vi "filter.post.state.vi"(11 "filter.data in":T1 {"memory.command"."order.slot.value"."Quantity" format="%016x"; "memory.command"."order.slot.value"."OrderId" format="%016x"; "memory.command"."ticker.slot.value"."Symbol" format="%016x"; "Scratch"."OrderId" format="%016x"}) -> (3 "filter.data out 2":T1 {"memory.command"."order.slot.value"."Quantity" format="%016x"; "memory.command"."order.slot.value"."OrderId" format="%016x"; "memory.command"."ticker.slot.value"."Symbol" format="%016x"; "Scratch"."OrderId" format="%016x"})   [LabVIEW 2022 SP3]
uses:
  filter.data.ctl
  filter.states.ctl
  filter.debug.ctl
  filter.debug.slot.ctl
  filter.data.scratch.ctl
  arty/orderbook/orderbook.command.ctl
  arty/orderbook/orderbook.command.type.ctl
  filter.memory.command.ctl
  ticker.slot.ctl
  order.slot.ctl
  <vilib>/rvi/DataTransferAndStorage/Container/Common/niFpgaContainerGetUniqueNameForEmu.vi
  <vilib>/rvi/DataTransferAndStorage/Container/Common/niFpgaContainerSetEmuInfo.vi
  <vilib>/rvi/eio/common/nirviEmuReportErrorAndStop.vi
  <vilib>/rvi/Emulation/niFpgaEmulationIsFPGAContextNoSignature.vi
  <vilib>/rvi/Emulation/niFpgaSctlEmulationGetInTimedLoop.vi
  <vilib>/rvi/errors/niFpgaSetErrorForExecOnDevCompSimple.vi
  <vilib>/rvi/FIFO/Fifo_Resource/nirvififoEmulationSetSize.vi
  <vilib>/rvi/FIFO/Fifo_Resource/nirviFifoEmulationQueueMgr.vi
  <instcachedir>/0/nirviFifoEmulationQueueMgr_E5CAEC123FF24DC58D834DCA3CDAA9B5.lvgen/nirviFifoEmulationQueueMgr_E5CAEC123FF24DC58D834DCA3CDAA9B5_017.vi
  <vilib>/rvi/FIFO/Fifo_Resource/nirvififoEmulationDetermineInputValidOut.vi
  <vilib>/rvi/FIFO/Fifo_Resource/nirvififoEmulationCreateLock.vi
  <vilib>/rvi/Emulation/niFpgaProcessEmulError.vi
  <vilib>/rvi/FIFO/Fifo_Resource/nirvififoEmulationObtainLock.vi
  <vilib>/rvi/FIFO/Fifo_Resource/nirvififoEmulationReleaseLock.vi
  <vilib>/rvi/occurrence/nirviWaitOnOccurrenceBase.vi
  <vilib>/rvi/errors/nirviReportUnexpectedCaseInternalError.vi
  <vilib>/rvi/errors/nirviReportUnexpectedCaseInternalError (U32).vi
  <instcachedir>/0/nirviFifoEmulationQueueMgr_E5CAEC123FF24DC58D834DCA3CDAA9B5.lvgen/nirviFifoEmulationQueueMgr_E5CAEC123FF24DC58D834DCA3CDAA9B5_011.vi
  <vilib>/rvi/DataTransferAndStorage/Container/Common/niFpgaContainerExecOnDevCompGetState.vi
  <vilib>/rvi/Memory/Memory_Emulation/niFpgaMemoryEmulationCacheClearOnFirstRun.vi
  <vilib>/rvi/Memory/Memory_Emulation/nirvimemoryEmulationManagerCache_MakeExclusive.vi
  <vilib>/rvi/Memory/Memory_Emulation/niFpgaMemoryEmulationValidateCache.vi
  <vilib>/rvi/Memory/Memory_Emulation/nirvimemoryEmulationManagerCache_InsertValue.vi
  <vilib>/Utility/error.llb/Clear Errors.vi
  <vilib>/rvi/Memory/Memory_Emulation/nirvimemoryEmulationManagerCache_ReleaseExclusive.vi
  <vilib>/rvi/Memory/Memory_Emulation/nirvimemoryEmulationManagerCache_GetValue.vi
  <vilib>/rvi/Memory/Memory_Emulation/nirvimemoryEmulationManagerCache_SetValue.vi
  <vilib>/rvi/Emulation/niFpgaSctlEmulationResourceMgr.vi
  <vilib>/rvi/LocalResourceManager/LocalResourceManager.xnode
  <vilib>/rvi/DataTransferAndStorage/Container/XNode/niFpgaContainer.xnode
  <vilib>/rvi/FIFO/Fifo_Resource/nirvififoEmulationWrite.vi
  <vilib>/rvi/Memory/Memory_Emulation/niFpgaMemoryEmulationRefIn.vi
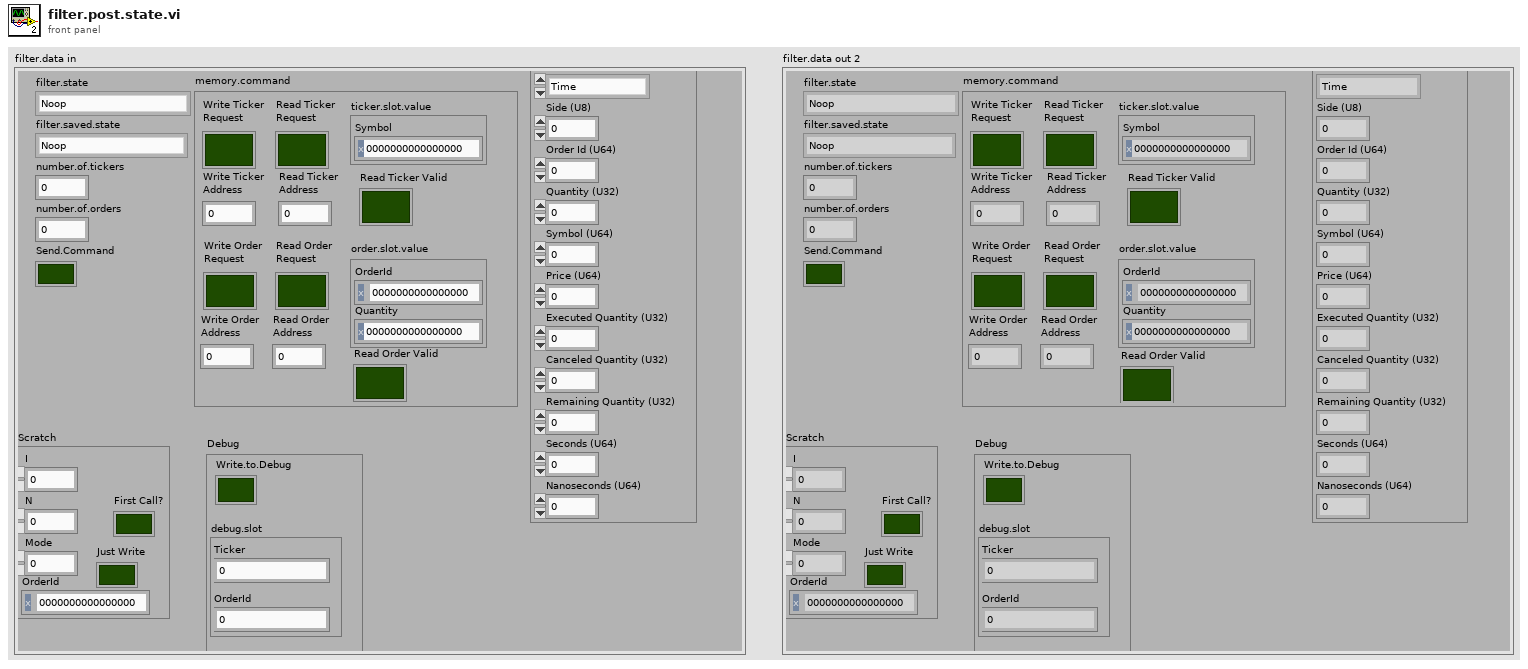
[diagram p1: front panel]
types:
  T1 = typedef "filter.data.ctl" = cluster{"filter.state":T2, "Debug":T3, "number.of.tickers":u32, "number.of.orders":u32, "filter.saved.state":T2, "Scratch":T5, "OrderBook.Command":T6, "Send.Command":bool, "memory.command":T8}
  T2 = typedef "filter.states.ctl" = enum16{"Noop", "Reset", "Debug", "Configuration", "Wait.for.Command", "Filter.Add", "Filter.Other", "Insert.Order", "Delete Order"}
  T3 = typedef "filter.debug.ctl" = cluster{"Write.to.Debug":bool, "debug.slot":T4}
  T4 = typedef "filter.debug.slot.ctl" = cluster{"Ticker":u64, "OrderId":u64}
  T5 = typedef "filter.data.scratch.ctl" = cluster{"I":u32, "N":u32, "Mode":u32, "OrderId":u64, "First Call?":bool, "Just Write":bool}
  T6 = typedef "orderbook.command.ctl" = cluster{"OrderBook Command.Type":T7, "Side (U8)":u8, "Order Id (U64)":u64, "Quantity (U32)":u32, "Symbol (U64)":u64, "Price (U64)":u64, "Executed Quantity (U32)":u32, "Canceled Quantity (U32)":u32, "Remaining Quantity (U32)":u32, "Seconds (U64)":u64, "Nanoseconds (U64)":u64}
  T7 = typedef "orderbook.command.type.ctl" = enum16{"Time", "AddOrder", "OrderExecuted", "OrderExecutedAtPrice", "ReduceSize", "ModifyOrder", "DeleteOrder", "Get.All.Orders", "Get.Top"}
  T8 = typedef "filter.memory.command.ctl" = cluster{"ticker.slot.value":T9, "order.slot.value":T10, "Write Ticker\nAddress":u32, "Write Ticker\nRequest":bool, "Read Ticker\nRequest":bool, "Read Ticker\nAddress":u32, "Read Ticker Valid":bool, "Write Order\nAddress":u32, "Write Order\nRequest":bool, "Read Order\nRequest":bool, "Read Order\nAddress":u32, "Read Order Valid":bool}
  T9 = typedef "ticker.slot.ctl" = cluster{"Symbol":u64}
  T10 = typedef "order.slot.ctl" = cluster{"OrderId":u64, "Quantity":u64}
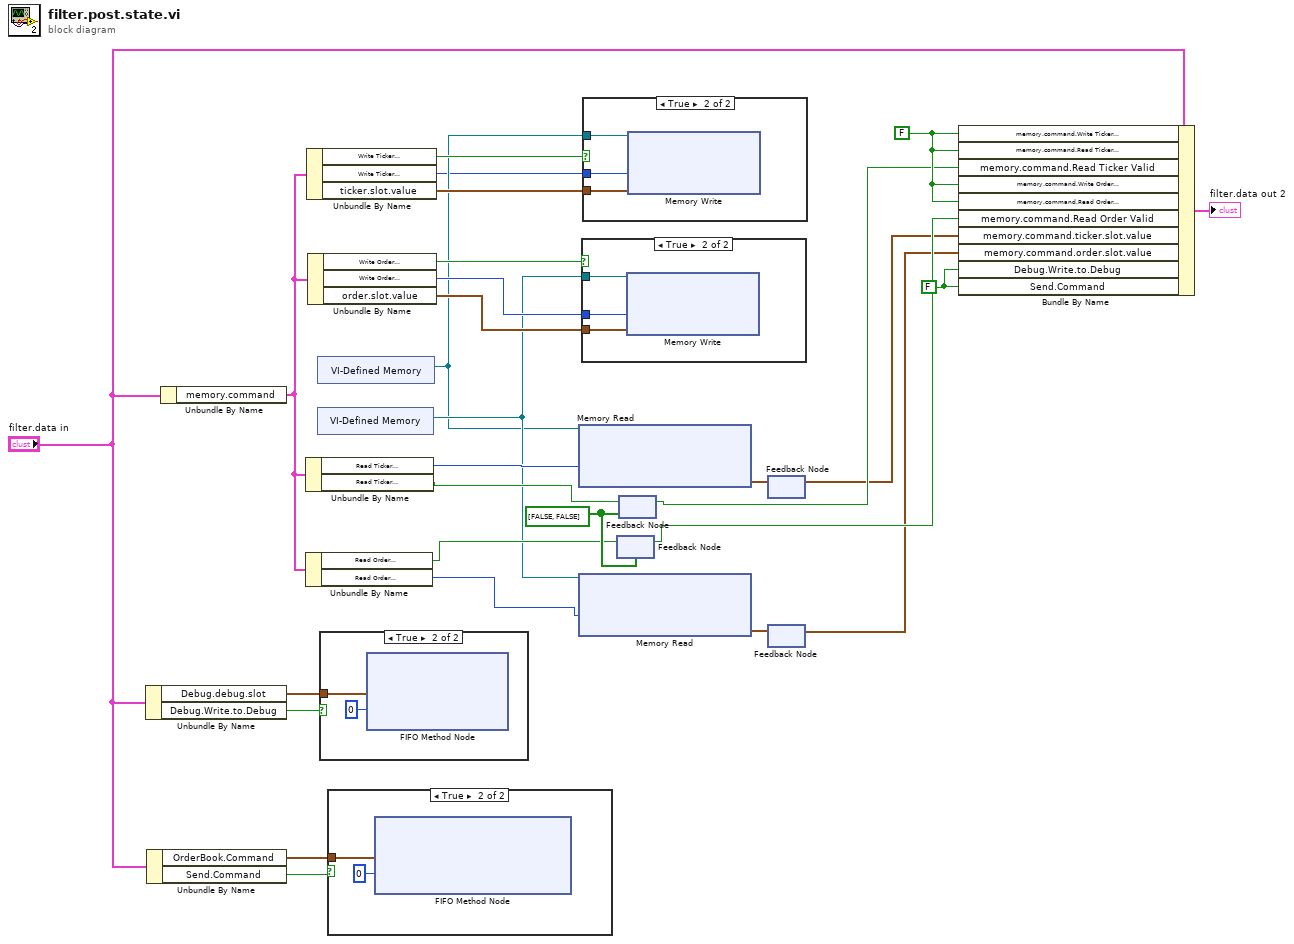
[diagram p0: block diagram]
diagram:
  w28 = FALSE ("memory.command.Write Ticker\nRequest")
  w25 = bool[] [FALSE, FALSE]
  w15 = FALSE ("Debug.Write.to.Debug")
  n1 = Unbundle By Name("filter.data in") -> ("Debug.debug.slot"=w11:T4, "Debug.Write.to.Debug"=w9:bool)
  n2 = Unbundle By Name("filter.data in") -> ("OrderBook.Command"=w14:T6, "Send.Command"=w13:bool)
  n3 = Unbundle By Name("filter.data in") -> ("memory.command"=w22:T8)
  n4 = Unbundle By Name(w22) -> ("Read Ticker\nAddress"=w4:u32, "Read Ticker\nRequest"=w21:bool)
  n5 = Unbundle By Name(w22) -> ("Read Order\nRequest"=w24:bool, "Read Order\nAddress"=w23:u32)
  n6 = Unbundle By Name(w22) -> ("Write Ticker\nRequest"=w16:bool, "Write Ticker\nAddress"=w1:u32, "ticker.slot.value"=w17:T9)
  n7 = Unbundle By Name(w22) -> ("Write Order\nRequest"=w18:bool, "Write Order\nAddress"=w19:u32, "order.slot.value"=w20:T10)
  n8 = xnode "VI-Defined Memory"() -> ("Memory Out"=w2:refnum<k21>)
  n9 = xnode "VI-Defined Memory"() -> ("Memory Out"=w3:refnum<k21>)
  n10 = case shown="True" w9 {
    tunnel: w11 -> [_ w30]
    frame False {
    }
    frame True {
      n11 = xnode ("FIFO Method Node")("Element"=w30, "Timeout"=0) -> ()  [unwired: 1 in, 2 out]
    }
  }
  n12 = case shown="True" w13 {
    tunnel: w14 -> [_ w31]
    frame False {
    }
    frame True {
      n13 = xnode ("FIFO Method Node")("Element"=w31, "Timeout"=0) -> ()  [unwired: 1 in, 2 out]
    }
  }
  n14 = xnode "Memory Read"("Address"=w4, "Memory In"=w2) -> ("Data"=w6:cluster{"Symbol":u64})  [unwired: 1 out]
  n15 = xnode "Memory Read"("Address"=w23, "Memory In"=w3) -> ("Data"=w5:cluster{"OrderId":u64, "Quantity":u64})  [unwired: 1 out]
  n16 = case shown="True" w18 {
    tunnel: w3 -> [_ w35]
    tunnel: w19 -> [_ w34]
    tunnel: w20 -> [_ w33]
    frame False {
    }
    frame True {
      n17 = xnode "Memory Write"("Address"=w34, "Data"=w33, "Memory In"=w35) -> ()  [unwired: 1 out]
    }
  }
  n18 = case shown="True" w16 {
    tunnel: w2 -> [_ w38]
    tunnel: w1 -> [_ w37]
    tunnel: w17 -> [_ w36]
    frame False {
    }
    frame True {
      n19 = xnode "Memory Write"("Address"=w37, "Data"=w36, "Memory In"=w38) -> ()  [unwired: 1 out]
    }
  }
  n20 = feedback #1(w25) -> (w27:bool)
  n21 = feedback-in #1(w24) -> ()
  n22 = feedback #2(w25) -> (w26:bool)
  n23 = feedback-in #2(w21) -> ()
  n24 = feedback #3() -> (w10:cluster{"Symbol":u64})  [unwired: 1 in]
  n25 = feedback-in #3(w6) -> ()
  n26 = feedback #4() -> (w8:cluster{"OrderId":u64, "Quantity":u64})  [unwired: 1 in]
  n27 = feedback-in #4(w5) -> ()
  n28 = Bundle By Name(cluster="filter.data in", "memory.command.Write Ticker\nRequest"=w28, "memory.command.Read Ticker\nRequest"=w28, "memory.command.Read Ticker Valid"=w26, "memory.command.Write Order\nRequest"=w28, "memory.command.Read Order\nRequest"=w28, "memory.command.Read Order Valid"=w27, "memory.command.ticker.slot.value"=w10, "memory.command.order.slot.value"=w8, "Debug.Write.to.Debug"=w15, "Send.Command"=w15) -> (→"filter.data out 2":T1)
